vi "Clad Exercise 3-6.vi"() -> ()   [LabVIEW 2014]
panel:
  in  "Kelvin":dbl
  in  "Celcius":dbl
  in  "Fahrenheit":dbl
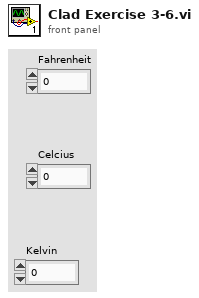
[diagram p1: front panel]
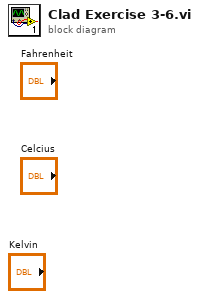
[diagram p0: block diagram]
diagram:
